vi "Inline - Update Error Counter Channel.vi"(6 "Inline Status Channels Refs":T1[](array[typedef]) format="%.0x", 8 "error in (no error)":errorcluster, 10 "Increment Unconfigured Frames Counter?":bool, 11 "error":u16) -> (0 "error IO":errorcluster, 3 "Hit":bool)   [LabVIEW 2017, in "Ballard MIL-1553 Engine.lvlib"]
uses:
  Ballard MIL-1553 Engine.lvlib
  <vilib>/NI Veristand/Custom Device API/Data Reference.ctl
  <vilib>/NI VeriStand/Custom Device API/Custom Device API.lvlib
panel:
  out "AnyError":bool
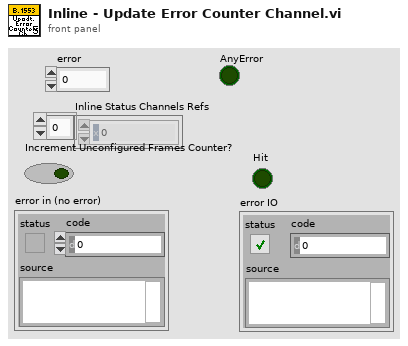
[diagram p1: front panel]
types:
  T1 = typedef "Custom Device API.lvlib/Data Reference.ctl" = i32
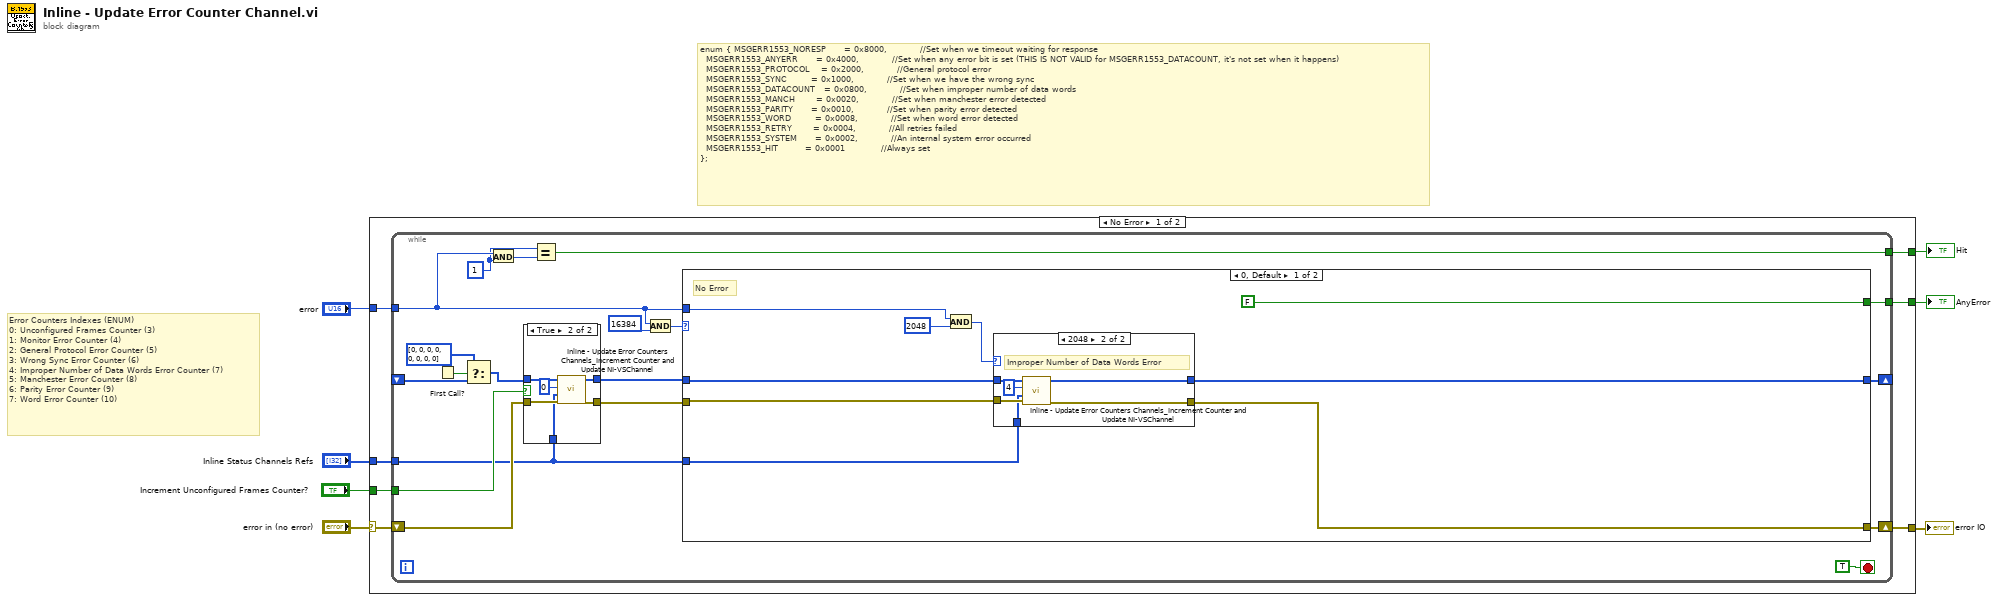
[diagram p0: block diagram]
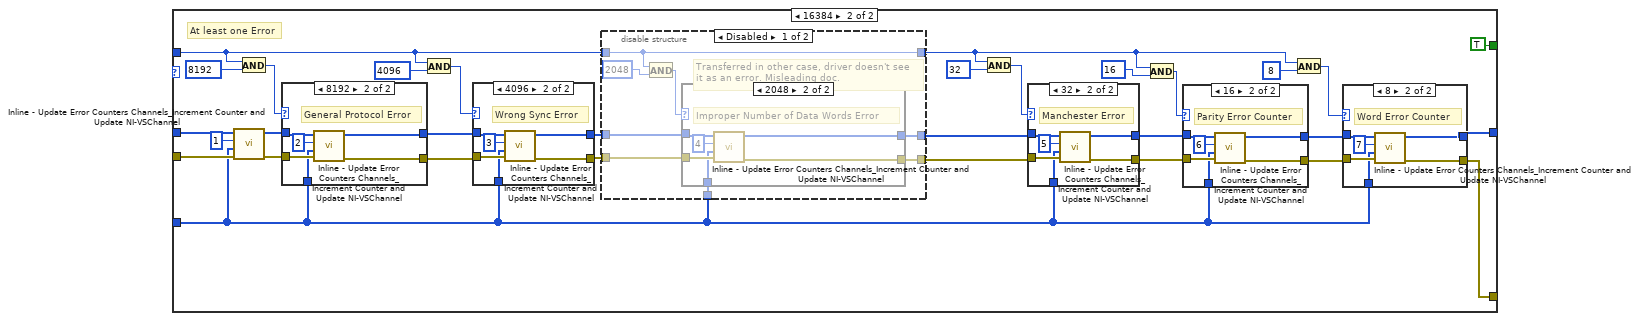
[diagram p4: hidden frame]
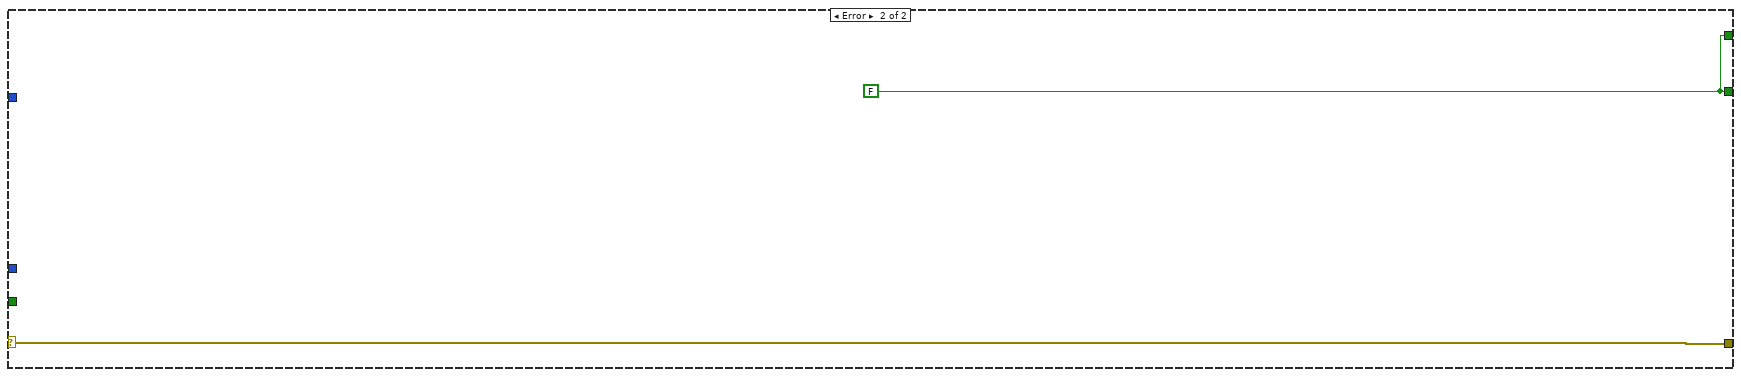
[diagram p12: hidden frame]
diagram:
  # "enum {\tMSGERR1553_NORESP      = 0x8000,           //Set when we timeout waiting for response\n\t\tMSGERR1553_ANYERR      = 0x4000,           //Set when any error bit is set (THIS IS NOT VALID for MSGERR1553_DATACOUNT, it's not set when it happens)  \n\t\tMSGERR1553_PROTOCOL    = 0x2000,           //General protocol error\n\t\tMSGERR1553_SYNC        = 0x1000,           //Set when we have the wrong sync\n\t\tMSGERR1553_DATACOUNT   = 0x0800,           //Set when improper number of data words\n\t\tMSGERR1553_MANCH       = 0x0020,           //Set when manchester error detected\n\t\tMSGERR1553_PARITY      = 0x0010,           //Set when parity error detected\n\t\tMSGERR1553_WORD        = 0x0008,           //Set when word error detected\n\t\tMSGERR1553_RETRY       = 0x0004,           //All retries failed\n\t\tMSGERR1553_SYSTEM      = 0x0002,           //An internal system error occurred\n\t\tMSGERR1553_HIT         = 0x0001            //Always set\n};"
  # "Error Counters Indexes (ENUM) \n0: Unconfigured Frames Counter (3)\n1: Monitor Error Counter (4)\n2: General Protocol Error Counter (5)\n3: Wrong Sync Error Counter (6)\n4: Improper Number of Data Words Error Counter (7)\n5: Manchester Error Counter (8)\n6: Parity Error Counter (9)\n7: Word Error Counter (10)"
  n1 = case shown="No Error" "error in (no error)" {
    selector: "error in (no error)" -> [w12 w150]
    tunnel: "Inline Status Channels Refs" -> [w14 _]
    tunnel: "error" -> [w13 _]
    tunnel: [w11 w150] -> w4
    tunnel: [w10 w149] -> w3
    tunnel: [w9 w149] -> w2
    tunnel: "Increment Unconfigured Frames Counter?" -> [w8 _]
    frame No Error {
      n2 = while {
        tunnel: w14 -> [w15]
        tunnel: w13 -> [w24]
        shift-right: [w31] -> w11
        shift-left: w12 -> [w17]
        shift-right: [w27] -> _
        shift-left: _ -> [w26]
        tunnel: [w25] -> w9
        tunnel: [w21] -> w10
        tunnel: w8 -> [w20]
        stop <- TRUE stop-if-true
        w22 = u16 1 ("y")
        n3 = First Call?() -> (First Call?: T/F=w29:bool)
        n4 = Select(t=u32[] [0, 0, 0, 0, 0, 0, 0, 0], s=w29, f=w26) -> (s? t:f=w19:u32[])
        n5 = And(x=w24, y=w22) -> (x .and. y?=w23:u16)
        n6 = case shown="True" w20 {
          tunnel: w19 -> [w35 w40]
          tunnel: [w35 w39] -> w18
          tunnel: w17 -> [w34 w41]
          tunnel: [w34 w38] -> w16
          tunnel: w15 -> [_ w37]
          frame False {
          }
          frame True {
            n7 = call "Inline - Update Error Counters Channels_Increment Counter and Update NI-VSChannel.vi"("error in (no error)"=w41, "Inline Status Channels Refs"=w37, "index"=0, "Error Counters Value In in"=w40) -> ("error out"=w38:errorcluster, "Error Counters Value In out"=w39:u32[])  [unwired: 6 in]
          }
        }
        n8 = Equal?(x=w22, y=w23) -> (x = y?=w21:bool)
        n9 = And(x=w24, y=u16 16384) -> (x .and. y?=w33:u16)
        n10 = case shown="0, Default" w33 {
          tunnel: w18 -> [w43 w89]
          tunnel: [w42 w63] -> w27
          tunnel: w15 -> [w44 w62]
          tunnel: w16 -> [w48 w87]
          tunnel: w24 -> [w46 w61]
          tunnel: [w47 w64] -> w31
          tunnel: [FALSE TRUE] -> w25
          frame 0, Default {
            # "No Error"
            n11 = And(x=w46, y=u16 2048) -> (x .and. y?=w45:u16)
            n12 = case shown="2048" w45 {
              tunnel: w48 -> [w52 w58]
              tunnel: [w51 w57] -> w42
              tunnel: [w52 w56] -> w47
              tunnel: w44 -> [_ w55]
              tunnel: w43 -> [w51 w53]
              frame 0, Default {
              }
              frame 2048 {
                # "Improper Number of Data Words Error"
                n13 = call "Inline - Update Error Counters Channels_Increment Counter and Update NI-VSChannel.vi"("error in (no error)"=w58, "Inline Status Channels Refs"=w55, "index"=4, "Error Counters Value In in"=w53) -> ("error out"=w56:errorcluster, "Error Counters Value In out"=w57:u32[])  [unwired: 6 in]
              }
            }
          }
          frame 16384 {
            # "At least one Error"
            n14 = call "Inline - Update Error Counters Channels_Increment Counter and Update NI-VSChannel.vi"("error in (no error)"=w87, "Inline Status Channels Refs"=w62, "index"=1, "Error Counters Value In in"=w89) -> ("error out"=w83:errorcluster, "Error Counters Value In out"=w84:u32[])  [unwired: 6 in]
            n15 = And(x=w61, y=u16 8192) -> (x .and. y?=w85:u16)
            n16 = case shown="8192" w85 {
              tunnel: w84 -> [w142 w147]
              tunnel: w83 -> [w141 w148]
              tunnel: [w142 w146] -> w80
              tunnel: [w141 w145] -> w79
              tunnel: w62 -> [_ w144]
              frame 0, Default {
              }
              frame 8192 {
                # "General Protocol Error"
                n17 = call "Inline - Update Error Counters Channels_Increment Counter and Update NI-VSChannel.vi"("error in (no error)"=w148, "Inline Status Channels Refs"=w144, "index"=2, "Error Counters Value In in"=w147) -> ("error out"=w145:errorcluster, "Error Counters Value In out"=w146:u32[])  [unwired: 6 in]
              }
            }
            n18 = And(x=w61, y=u16 4096) -> (x .and. y?=w81:u16)
            n19 = case shown="4096" w81 {
              tunnel: w80 -> [w134 w139]
              tunnel: w79 -> [w133 w140]
              tunnel: [w134 w138] -> w78
              tunnel: [w133 w137] -> w77
              tunnel: w62 -> [_ w136]
              frame 0, Default {
              }
              frame 4096 {
                # "Wrong Sync Error"
                n20 = call "Inline - Update Error Counters Channels_Increment Counter and Update NI-VSChannel.vi"("error in (no error)"=w140, "Inline Status Channels Refs"=w136, "index"=3, "Error Counters Value In in"=w139) -> ("error out"=w137:errorcluster, "Error Counters Value In out"=w138:u32[])  [unwired: 6 in]
              }
            }
            n21 = disable-structure shown="Disabled" {
              disable-tunnel: w78 -> [w96 w107]
              disable-tunnel: w77 -> [w95 w108]
              disable-tunnel: [w93 w107] -> w76
              disable-tunnel: [w92 w108] -> w75
              disable-tunnel: w62 -> [w91 _]
              disable-tunnel: w61 -> [w90 w106]
              disable-tunnel: [w90 w106] -> w59
              frame Disabled {
                # "Transferred in other case, driver doesn't see\nit as an error. Misleading doc."
                n22 = And(x=w90, y=u16 2048) -> (x .and. y?=w94:u16)
                n23 = case shown="2048" w94 {
                  tunnel: w96 -> [w99 w104]
                  tunnel: w95 -> [w98 w105]
                  tunnel: [w99 w103] -> w93
                  tunnel: [w98 w102] -> w92
                  tunnel: w91 -> [_ w101]
                  frame 0, Default {
                  }
                  frame 2048 {
                    # "Improper Number of Data Words Error"
                    n24 = call "Inline - Update Error Counters Channels_Increment Counter and Update NI-VSChannel.vi"("error in (no error)"=w105, "Inline Status Channels Refs"=w101, "index"=4, "Error Counters Value In in"=w104) -> ("error out"=w102:errorcluster, "Error Counters Value In out"=w103:u32[])  [unwired: 6 in]
                  }
                }
              }
              frame Enabled {
              }
            }
            n25 = And(x=w59, y=u16 32) -> (x .and. y?=w73:u16)
            n26 = case shown="32" w73 {
              tunnel: w76 -> [w126 w131]
              tunnel: w75 -> [w125 w132]
              tunnel: [w126 w130] -> w66
              tunnel: [w125 w129] -> w65
              tunnel: w62 -> [_ w128]
              frame 0, Default {
              }
              frame 32 {
                # "Manchester Error"
                n27 = call "Inline - Update Error Counters Channels_Increment Counter and Update NI-VSChannel.vi"("error in (no error)"=w132, "Inline Status Channels Refs"=w128, "index"=5, "Error Counters Value In in"=w131) -> ("error out"=w129:errorcluster, "Error Counters Value In out"=w130:u32[])  [unwired: 6 in]
              }
            }
            n28 = And(x=w59, y=u16 16) -> (x .and. y?=w67:u16)
            n29 = case shown="16" w67 {
              tunnel: w66 -> [w118 w123]
              tunnel: w65 -> [w117 w124]
              tunnel: [w118 w122] -> w68
              tunnel: [w117 w121] -> w69
              tunnel: w62 -> [_ w120]
              frame 0, Default {
              }
              frame 16 {
                # "Parity Error Counter"
                n30 = call "Inline - Update Error Counters Channels_Increment Counter and Update NI-VSChannel.vi"("error in (no error)"=w124, "Inline Status Channels Refs"=w120, "index"=6, "Error Counters Value In in"=w123) -> ("error out"=w121:errorcluster, "Error Counters Value In out"=w122:u32[])  [unwired: 6 in]
              }
            }
            n31 = And(x=w59, y=u16 8) -> (x .and. y?=w71:u16)
            n32 = case shown="8" w71 {
              tunnel: w68 -> [w110 w115]
              tunnel: w69 -> [w109 w116]
              tunnel: [w110 w114] -> w63
              tunnel: [w109 w113] -> w64
              tunnel: w62 -> [_ w112]
              frame 0, Default {
              }
              frame 8 {
                # "Word Error Counter"
                n33 = call "Inline - Update Error Counters Channels_Increment Counter and Update NI-VSChannel.vi"("error in (no error)"=w116, "Inline Status Channels Refs"=w112, "index"=7, "Error Counters Value In in"=w115) -> ("error out"=w113:errorcluster, "Error Counters Value In out"=w114:u32[])  [unwired: 6 in]
              }
            }
          }
        }
      }
    }
    frame Error {
      w149 = FALSE
    }
  }
  "error IO" <- w4
  "Hit" <- w3
  "AnyError" <- w2
